vi "RFmx_OneShot_Test.vi"() -> ()   [LabVIEW 2014]
uses:
  <vilib>/RFmx/SpecAn/mx/RFmxSpecAn.llb/RFmxSpecAn Configure Digital Edge Trigger.vi
  <vilib>/RFmx/SpecAn/mx/RFmxSpecAn.llb/RFmxSpecAn Select Measurement (Multiple).vi
panel:
  in  "Stop Button":bool
  out "Results":string="ACP : -20.73\r\nCHP : -20.73\r\nTXP : -36.22\r\n"
  in  "RFmx_Setting":T1={"Center Frequency (Hz)"=1150000000.0, "Reference Level (dBm)"=-15.0, "External Attenuation (dB)"=0.0, "ACP:Offset Frequency (Hz)"=[5000000.0, 10000000.0, 12500000.0], "ACP:Integration Bandwidth (Hz)"=[9000000.0, 9000000.0, 9000000.0], "CCDF:Threshold Level (dB or dBm)"=0.0, "CHP:Integration Bandwidth (Hz)"=9000000.0, "Fcnt:Threshold Level (dB or dBm)"=0.0, "OBW:Bandwidth Percentage (%)"=0.0, "Spectrum:Span (Hz)"=20000000.0, "TXP:Measurement Interval (s)"=0.1, "IQ:Bandwidth (Hz)"=1000000.0} {"IQ:Bandwidth (Hz)" format="%#_13p"; "TXP:Measurement Interval (s)" format="%#_6p"; "Spectrum:Span (Hz)" format="%#_13p"; "OBW:Bandwidth Percentage (%)" format="%#_6p"; "Fcnt:Threshold Level (dB or dBm)" format="%#_6p"; "CHP:Integration Bandwidth (Hz)" format="%#_6p"; "CCDF:Threshold Level (dB or dBm)" format="%#_6p"; "ACP:Integration Bandwidth (Hz)" format="%#_6p"; "ACP:Offset Frequency (Hz)" format="%#_6p"; "External Attenuation (dB)" format="%#_6p"; "Reference Level (dBm)" format="%#_6p"; "Center Frequency (Hz)" format="%#_6p"}
  out "x-y":dbl=0.27257474641373847
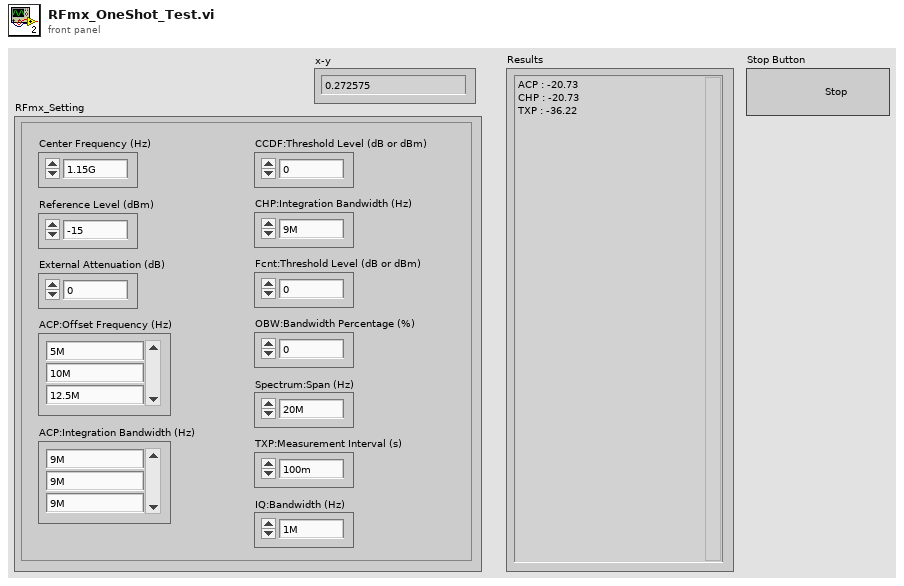
[diagram p1: front panel]
types:
  T1 = cluster{"Center Frequency (Hz)":dbl, "Reference Level (dBm)":dbl, "External Attenuation (dB)":dbl, "ACP:Offset Frequency (Hz)":dbl[], "ACP:Integration Bandwidth (Hz)":dbl[], "CCDF:Threshold Level (dB or dBm)":dbl, "CHP:Integration Bandwidth (Hz)":dbl, "Fcnt:Threshold Level (dB or dBm)":dbl, "OBW:Bandwidth Percentage (%)":dbl, "Spectrum:Span (Hz)":dbl, "TXP:Measurement Interval (s)":dbl, "IQ:Bandwidth (Hz)":dbl}
  T2 = enum16{"ACP", "CCDF", "CHP", "FCnt", "Harmonics", "OBW", "SEM", "Spectrum", "Spur", "TXP", "AMPM", "DPD", "IQ"}[]
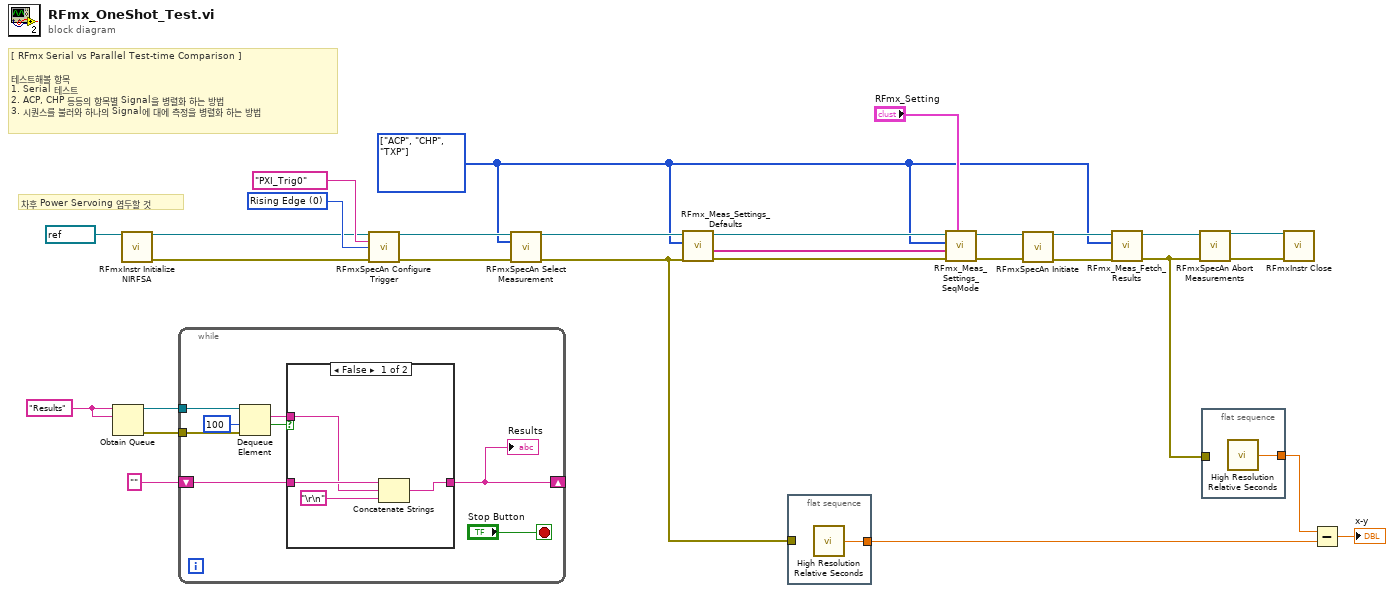
[diagram p0: block diagram]
diagram:
  w11 = "Results" ("name (unnamed)")
  w5 = T2 [enum."ACP", enum."CHP", enum."TXP"] items=["ACP", "CCDF", "CHP", "FCnt", "Harmonics", "OBW", "SEM", "Spectrum", "Spur", "TXP", "AMPM", "DPD", "IQ"] ("Measurements")
  w27 = 0 items=["Rising Edge", "Falling Edge"] ("Digital Edge")
  # "차후 Power Servoing 염두할 것"
  # "[ RFmx Serial vs Parallel Test-time Comparison ]\n\n테스트해볼 항목\n1. Serial 테스트\n2. ACP, CHP 등등의 항목별 Signal을 병렬화 하는 방법\n3. 시퀀스를 불러와 하나의 Signal에 대에 측정을 병렬화 하는 방법"
  n1 = Obtain Queue(name (unnamed)=w11, element data type=w11) -> (queue out=w10:refnum<queue>, error out=w9:errorcluster)  [unwired: 3 in, 1 out]
  n2 = call <vilib>:"RFmxInstr Initialize NIRFSA.vi"("Resource Name"=refnum<k15> "VST") -> ("Instrument Handle Out"=w19:refnum<k21>, "error out"=w18:errorcluster)  [unwired: 12 in, 1 out]
  n3 = while {
    tunnel: w10 -> [w37]
    tunnel: w9 -> [w36]
    shift-right: [w32] -> _
    shift-left: "" -> [w33]
    stop <- "Stop Button" stop-if-true
    n4 = Dequeue Element(queue=w37, timeout in ms (-1)=100, error in (no error)=w36) -> (element=w34:string, timed out?=w35:bool)  [unwired: 2 out]
    n5 = case shown="False" w35 {
      tunnel: w34 -> [w40 _]
      tunnel: w33 -> [w41 w42]
      tunnel: [w39 w42] -> w32
      frame False {
        n6 = Concatenate Strings(w41, w40, "\r\n") -> (w39:string)
      }
      frame True {
      }
    }
    "Results" <- w32
  }
  n7 = call-poly <vilib>:"RFmxSpecAn Configure Trigger.vi"("Instrument Handle In"=w19, "Digital Edge Source"="PXI_Trig0", "Digital Edge"=w27, "error in (no error)"=w18) -> ("Instrument Handle Out"=w26:refnum<k21>, "error out"=w25:errorcluster)  [unwired: 10 in]
  n8 = call-poly <vilib>:"RFmxSpecAn Select Measurement.vi"("Instrument Handle In"=w26, "Measurements"=w5, "error in (no error)"=w25) -> ("Instrument Handle Out"=w24:refnum<k21>, "error out"=w20:errorcluster)  [unwired: 11 in]
  n9 = call "RFmx_Meas_Settings_Defaults.vi"("error in"=w20, "Measurements"=w5, "Instrument Handle in"=w24) -> ("error out"=w16:errorcluster, "Selector_Strings"=w15:string[], "Instrument Handle out"=w17:refnum<k21>)  [unwired: 6 in]
  n10 = flat-sequence {
    tunnel: w20 -> [_]
    tunnel: [w43] -> w22
    frame #0 {
      n11 = call <vilib>:"High Resolution Relative Seconds.vi"() -> ("relative seconds"=w43:dbl)
    }
  }
  n12 = call "RFmx_Meas_Settings_SeqMode.vi"("RFmx_Setting"="RFmx_Setting", "error in"=w16, "Selector Strings"=w15, "Measurements"=w5, "Instrument Handle in"=w17) -> ("error out"=w12:errorcluster, "Instrument Handle out"=w13:refnum<k21>)  [unwired: 5 in]
  n13 = call <vilib>:"RFmxSpecAn Initiate.vi"("Instrument Handle In"=w13, "error in (no error)"=w12) -> ("Instrument Handle Out"=w7:refnum<k21>, "error out"=w6:errorcluster)  [unwired: 11 in, 1 out]
  n14 = call "RFmx_Meas_Fetch_Results.vi"("error in"=w6, "Measurements"=w5, "Instrument Handle in"=w7) -> ("error out"=w1:errorcluster, "Instrument Handle out"=w4:refnum<k21>)  [unwired: 7 in]
  n15 = call <vilib>:"RFmxSpecAn Abort Measurements.vi"("Instrument Handle In"=w4, "error in (no error)"=w1) -> ("Instrument Handle Out"=w2:refnum<k21>, "error out"=w3:errorcluster)  [unwired: 12 in]
  n16 = flat-sequence {
    tunnel: [w44] -> w23
    tunnel: w1 -> [_]
    frame #0 {
      n17 = call <vilib>:"High Resolution Relative Seconds.vi"() -> ("relative seconds"=w44:dbl)
    }
  }
  n18 = call <vilib>:"RFmxInstr Close.vi"("Instrument Handle In"=w2, "error in (no error)"=w3) -> ()  [unwired: 13 in, 1 out]
  n19 = Subtract(x=w23, y=w22) -> (x-y=→"x-y":dbl)
